vi "um2volts.vi"(7 "Kxyz":cluster{"Kx":dbl, "Ky":dbl, "Kz":dbl}, 9 "dxyz":cluster{"dx":dbl, "dy":dbl, "dz":dbl}) -> (2 "Vxyz":cluster{"Vx":dbl, "Vy":dbl, "Vz":dbl})   [LabVIEW 2014]
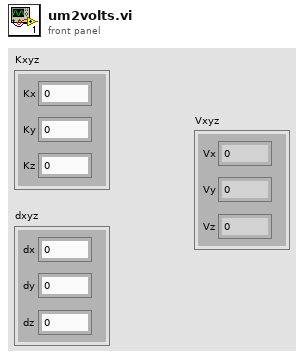
[diagram p1: front panel]
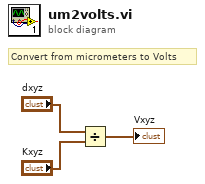
[diagram p0: block diagram]
diagram:
  # "Convert from micrometers to Volts"
  n1 = Divide(x="dxyz", y="Kxyz") -> (x/y=→"Vxyz":cluster{dbl, dbl, dbl})
